vi "Load Config.vi"(6 "Constants":refnum<class "Sequence Constants.lvclass">, 8 "error in (no error)":refnum<class "MultiErrors.lvclass">, 10 "Config Element":refnum<class "Config Element.lvclass">, 11 "SeqLoaded Condition Config in":refnum<class "SeqLoaded Condition Config.lvclass">) -> (0 "error out":refnum<class "MultiErrors.lvclass">, 3 "SeqLoaded Condition Config out":refnum<class "SeqLoaded Condition Config.lvclass">)   [LabVIEW 2020, in "VolatusSeqConfig.lvlib" / "SeqLoaded Condition Config.lvclass"]
uses:
  SeqLoaded Condition Config.lvclass
  VolatusErrorUtilities/MultiErrors/MultiErrors.lvclass
  lv-cdm/CDM-Config/Config Element/Config Element.lvclass
  SeqLoaded Condition Config.lvclass/SeqLoaded Condition Config.ctl
  Sequence Constants/Sequence Constants.lvclass
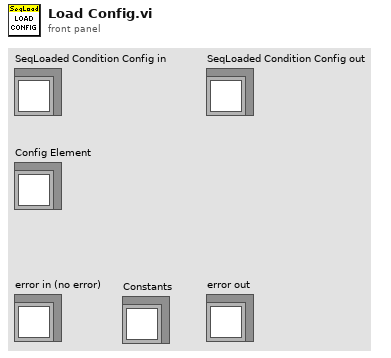
[diagram p1: front panel]
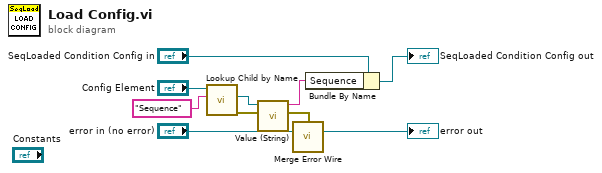
[diagram p0: block diagram]
diagram:
  n1 = call "Lookup Child by Name.vi"("Name"="Sequence", "Config Element in"="Config Element") -> ("error out"=w7:errorcluster, "Child"=w6:refnum<class "Config Element.lvclass">)  [unwired: 6 in, 2 out]
  n2 = call "Value (String).vi"("error in (no error)"=w7, "Config Element in"=w6) -> ("error out"=w2:errorcluster, "String Value"=w4:string)  [unwired: 8 in]
  n3 = call "Merge Error Wire.vi"("error in (no error)"=w2, "MultiErrors in"="error in (no error)") -> ("MultiErrors out"=→"error out":refnum<class "MultiErrors.lvclass">)  [unwired: 13 in]
  n4 = Bundle By Name(cluster="SeqLoaded Condition Config in", "Sequence"=w4) -> (→"SeqLoaded Condition Config out":refnum<class "SeqLoaded Condition Config.lvclass">)
